vi "RadsLeft.vi"(9 "dt":dbl, 10 "Cw2":dbl, 11 "Cw1":dbl) -> (3 "Rs":dbl)   [LabVIEW 2016]
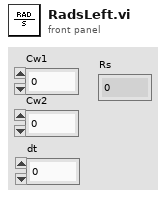
[diagram p1: front panel]
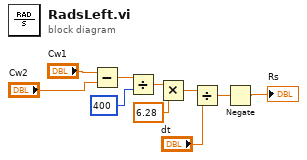
[diagram p0: block diagram]
diagram:
  n1 = Subtract(x="Cw1", y="Cw2") -> (x-y=w10:dbl)
  n2 = Divide(x=w10, y=400) -> (x/y=w8:dbl)
  n3 = Multiply(x=w8, y=6.28) -> (x*y=w6:dbl)
  n4 = Divide(x=w6, y="dt") -> (x/y=w2:dbl)
  n5 = Negate(x=w2) -> (-x=→"Rs":dbl)
